vi "terminate.vi"(8 "error in (no error)":errorcluster, 11 "DL090603DAQmxOnOffEmissionSensor in":refnum<class "DetectorDL090603DAQmxOnOff.lvclass">=refnum) -> (0 "error out":errorcluster, 3 "DL090603DAQmxOnOffEmissionSensor out":refnum<class "DetectorDL090603DAQmxOnOff.lvclass">)   [LabVIEW 2010, in "DetectorDL090603DAQmxOnOff.lvclass"]
doc: "The dynamic dispatch version of this VI terminates the plug-in object by releasing all of its resources."
uses:
  DetectorDL090603DAQmxOnOff.lvclass
  DetectorDL090603DAQmxOnOff.lvclass/DetectorDL090603DAQmxOnOff.ctl
  DigitalOut/DigitalOutDL110325DAQmx/DigitalOutDL110325DAQmx/DigitalOutDL110325DAQmx.lvclass
  GenericDetector/GenericDetector/GenericDetector.lvclass
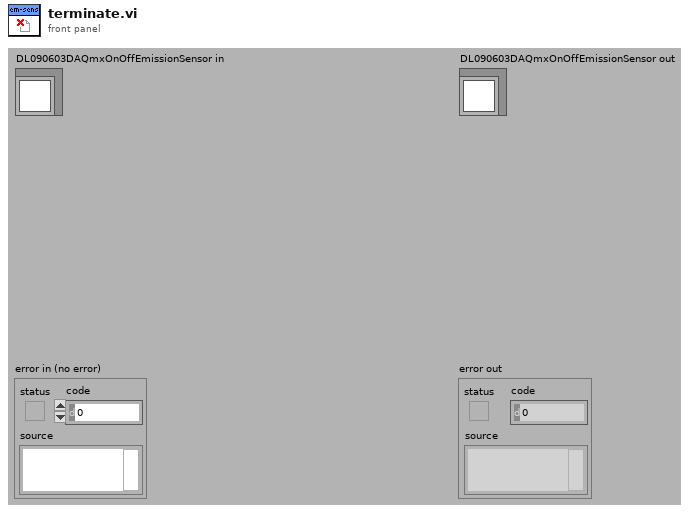
[diagram p1: front panel]
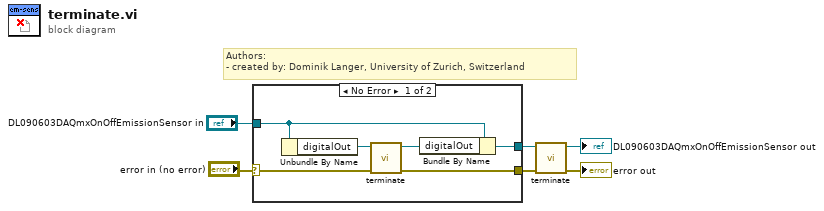
[diagram p0: block diagram]
diagram:
  # "Authors: \n- created by: Dominik Langer, University of Zurich, Switzerland"
  n1 = case shown="No Error" "error in (no error)" {
    selector: "error in (no error)" -> [w11 w14]
    tunnel: "DL090603DAQmxOnOffEmissionSensor in" -> [w8 w13]
    tunnel: [w12 w13] -> w3
    tunnel: [w7 w14] -> w4
    frame No Error {
      n2 = Unbundle By Name(w8) -> ("digitalOut"=w10:refnum<class "DigitalOutDL110325DAQmx.lvclass">)
      n3 = call-dynamic "terminate.vi"("error in (no error)"=w11, "DAQmxDigitalOut in"=w10) -> ("error out"=w7:errorcluster, "DAQmxDigitalOut out"=w9:refnum<class "DigitalOutDL110325DAQmx.lvclass">)  [unwired: 8 out]
      n4 = Bundle By Name(cluster=w8, "digitalOut"=w9) -> (w12:refnum<class "DetectorDL090603DAQmxOnOff.lvclass">)
    }
    frame Error {
    }
  }
  n5 = call-parent "terminate.vi"("error in (no error)"=w4, "GenericPlugin in"=w3) -> ("error out"=→"error out":errorcluster, "GenericPlugin out"=→"DL090603DAQmxOnOffEmissionSensor out":refnum<class "DetectorDL090603DAQmxOnOff.lvclass">)  [unwired: 8 out]
